vi "Channel path to TDMS Group and Channel.vi"(11 "Channel Path":string) -> (2 "TDMS Channel":string, 3 "TDMS Group":string)   [LabVIEW 2011]
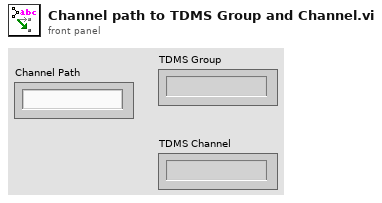
[diagram p1: front panel]
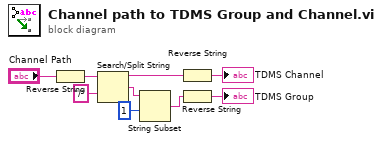
[diagram p0: block diagram]
diagram:
  n1 = Reverse String(1:"Channel Path") -> (0:w8:string)
  n2 = Search/Split String(string=w8, search string/char (-)="/") -> (substring before match=w6:string, match + rest of string=w3:string)  [unwired: 1 in, 1 out]
  n3 = String Subset(string=w3, offset (0)=1) -> (substring=w1:string)  [unwired: 1 in]
  n4 = Reverse String(1:w6) -> (0:→"TDMS Channel":string)
  n5 = Reverse String(1:w1) -> (0:→"TDMS Group":string)
